vi "Linear curve.vi"(1 "Orientation":enum16{"Horizontal", "Vertical"}(ring), 2 "Input X or Y Value":dbl, 3 "Point 2":cluster{"X":dbl, "Y":dbl}, 4 "Point 1":cluster{"X":dbl, "Y":dbl}) -> (0 "Output Value":dbl)   [LabVIEW 2011]
doc: "This VI uses the point-slope formula to fit an X or Y value to a linear curve."
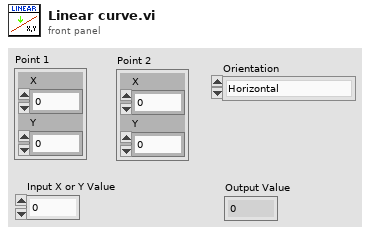
[diagram p1: front panel]
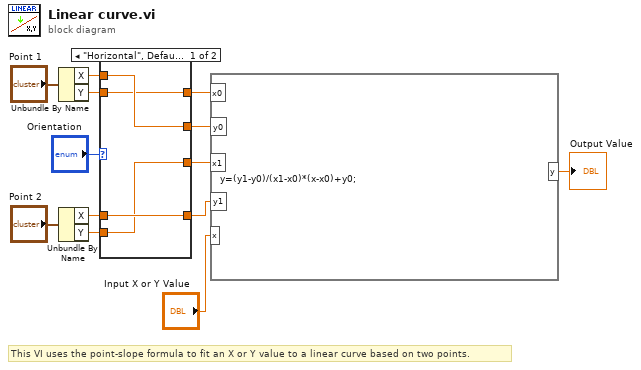
[diagram p0: block diagram]
diagram:
  # "This VI uses the point-slope formula to fit an X or Y value to a linear curve based on two points."
  n1 = Unbundle By Name("Point 1") -> ("X"=w8:dbl, "Y"=w7:dbl)
  n2 = Unbundle By Name("Point 2") -> ("X"=w6:dbl, "Y"=w5:dbl)
  n3 = case shown="\"Horizontal\", Default" "Orientation" {
    tunnel: w8 -> [w17 w18]
    tunnel: w7 -> [w16 w19]
    tunnel: w6 -> [w15 w20]
    tunnel: w5 -> [w14 w21]
    tunnel: [w16 w18] -> w4
    tunnel: [w17 w19] -> w3
    tunnel: [w14 w20] -> w2
    tunnel: [w15 w21] -> w1
    frame "Horizontal", Default {
    }
    frame "Vertical" {
    }
  }
  n4 = formula code="y=(y1-y0)/(x1-x0)*(x-x0)+y0;"("x0"=w4, "y0"=w3, "x1"=w2, "y1"=w1, "x"="Input X or Y Value") -> ("y"=→"Output Value":dbl)
